vi "HitrapGUI.HTLE_Main.vi"() -> ()   [LabVIEW 2014, in "HitrapGUI.lvlib"]
uses:
  HitrapGUI.lvlib
  CSlibraries/GUILib/GUILib.userEventsMainType.ctl
  CSlibraries-extern/DimLVEvent/DimIndicators/DimIndicators.anyType.ctl
  CSlibraries/UtilityLib/UtilityLib.lvlib
  CSlibraries-extern/DimLVEvent/DimIndicators/DimIndicators.lvlib
  CS_Core/CSSystem/CSSystemLib/CSSystemLib.lvlib
  CS_Core/GUIs/GOGControllerGUI/GOGControllerGUI.lvlib
  CSlibraries/GUILib/GUILib.lvlib
panel:
  in  "TR7":bool
  out "subSystem6State":string
  out "subSystem6StateQuality":string
  in  "TR6-UpperPart":bool
  in  "TR6-LowerPart":bool
  out "subSystem5State":string
  out "subSystem5StateQuality":string
  out "subSystem4State":string
  out "subSystem4StateQuality":string
  in  "TR6BT1":bool
  out "subSystem3State":string
  out "subSystem3StateQuality":string
  in  "TR5":bool
  out "subSystem2State":string
  out "subSystem2StateQuality":string
  in  "NoGUI":bool
  out "subSystem1State":string
  out "subSystem1StateQuality":string
  in  "iniData":string
  in  "subControllersIgnoredDIM":T1
  in  "stop":bool
  in  "userEvent":refnum<user-event>
  # "HITRAP_LE"
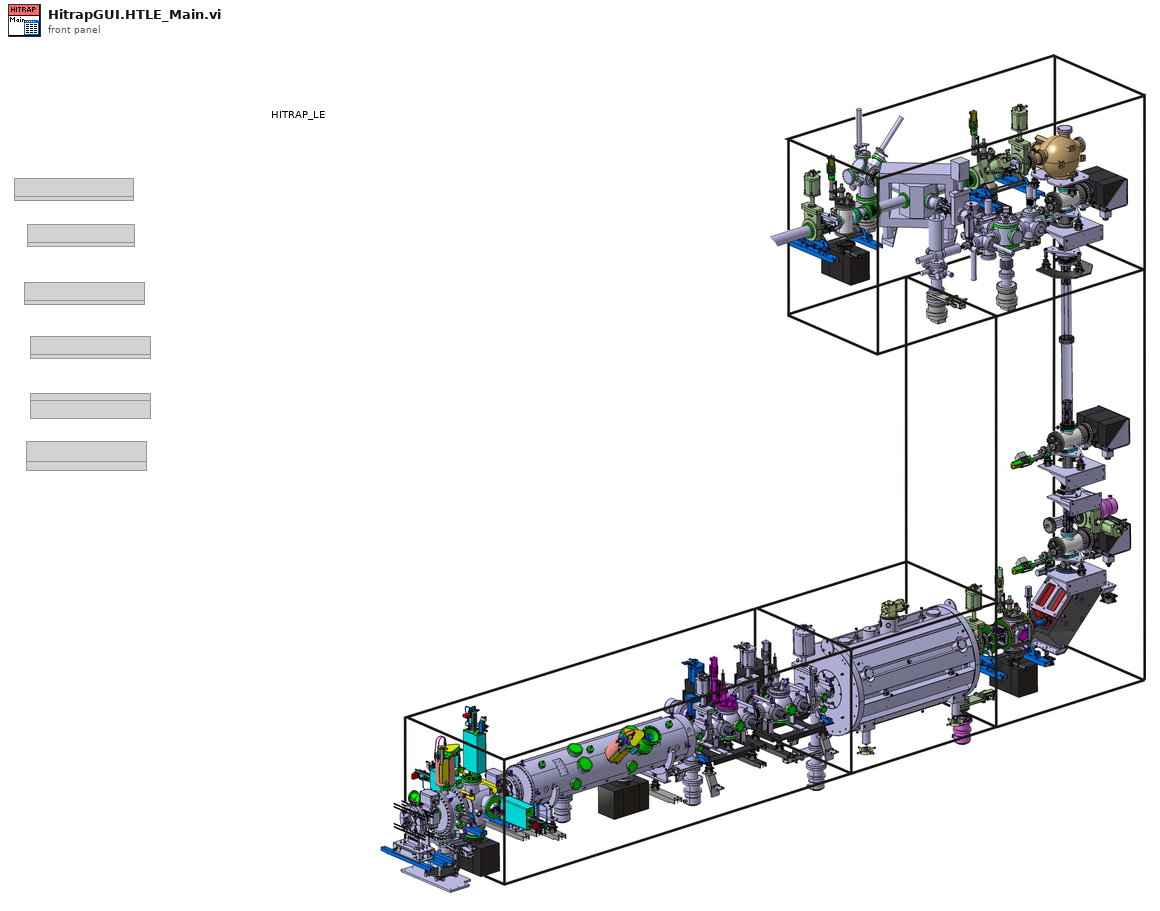
[diagram p1: front panel]
types:
  T1 = typedef "DimIndicators.lvlib/DimIndicators.anyType.ctl" = cluster{"data":string, "no link":bool, "quality":i32, "timeStamp":dbl}
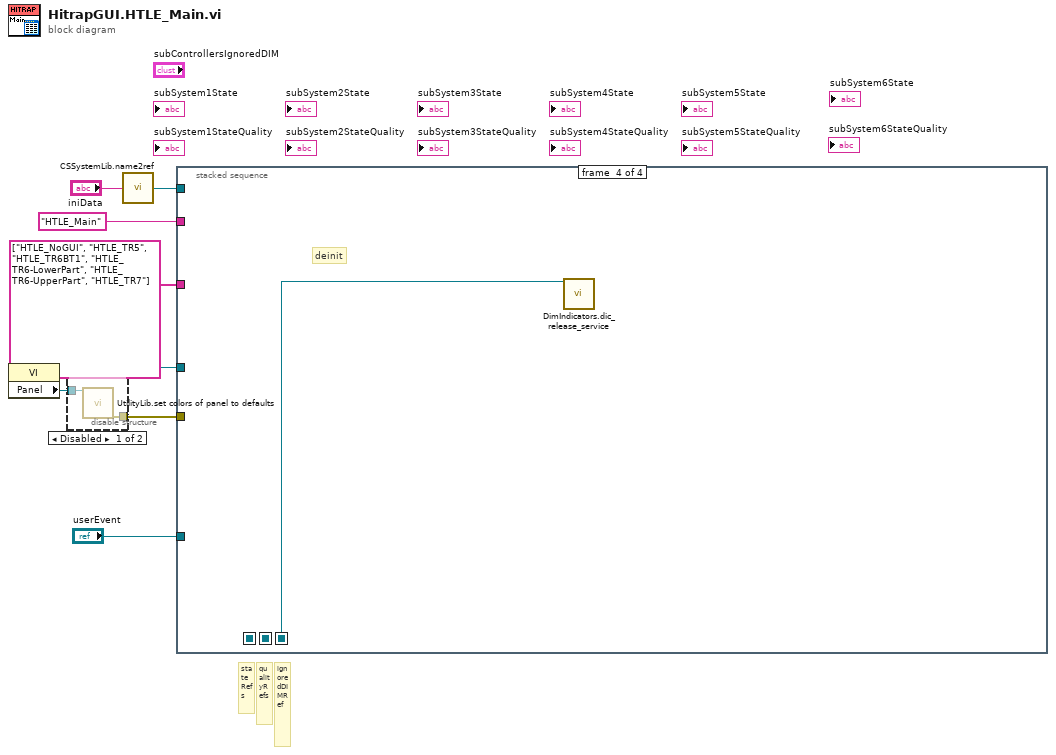
[diagram p0: block diagram]
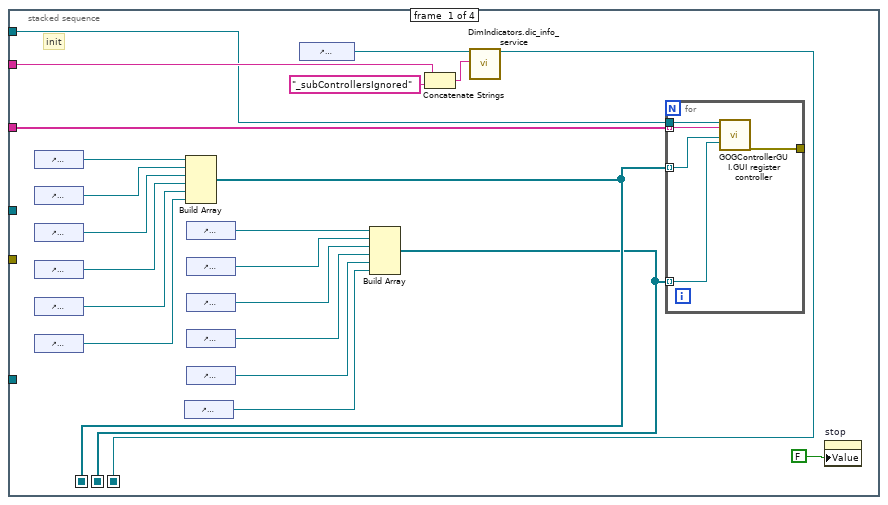
[diagram p3: hidden frame]
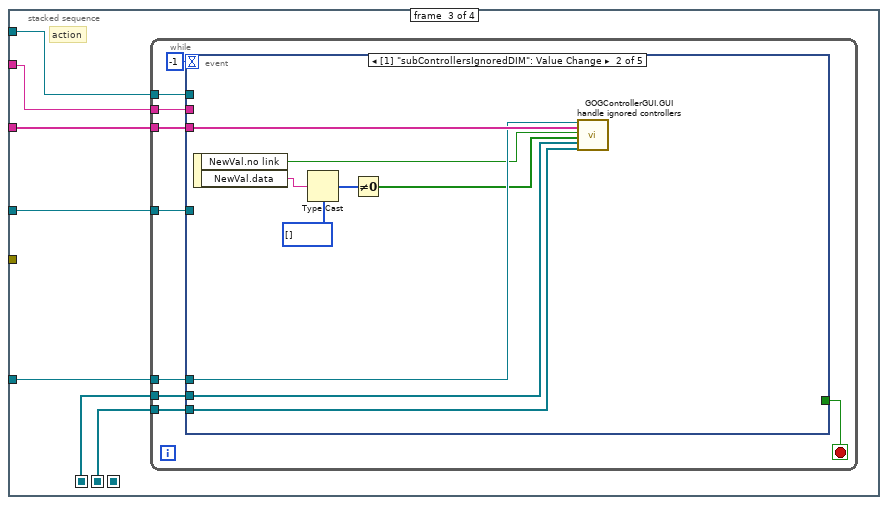
[diagram p5: hidden frame]
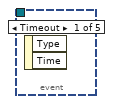
[diagram p6: hidden frame]
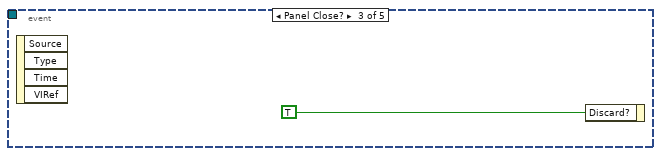
[diagram p7: hidden frame]
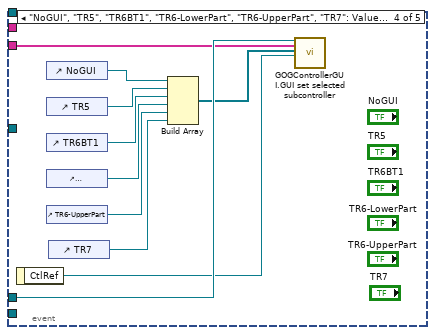
[diagram p8: hidden frame]
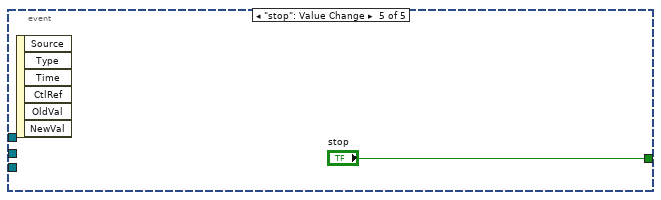
[diagram p9: hidden frame]
diagram:
  # "qualityRefs"
  # "ignoredDIMRef"
  # "stateRefs"
  n1 = property class="VI"() -> (reference out=w6:refnum<vi>, "Panel"=w7:refnum<vi>)  [unwired: 2 in, 1 out]
  n2 = disable-structure shown="Disabled" {
    disable-tunnel: w7 -> [w10 _]
    disable-tunnel: [w9 _] -> w4
    frame Disabled {
      n3 = call "UtilityLib.set colors of panel to defaults.vi"("Front Panel"=w10) -> ("error out"=w9:errorcluster)  [unwired: 18 in]
    }
    frame Enabled {
    }
  }
  n4 = call "CSSystemLib.name2ref.vi"("name"="iniData") -> ("obj refnum"=w1:refnum<vi>)
  n5 = stacked-sequence {
    seq-local: [w25 _ _ _] -> [_ _ _ w75]
    seq-local: [w26 _ _ _] -> [_ _ w41 _]
    seq-local: [w21 _ _ _] -> [_ _ w38 _]
    tunnel: "userEvent" -> [_ _ w44 _]
    tunnel: w6 -> [_ _ w43 _]
    tunnel: string[] ["HTLE_NoGUI", "HTLE_TR5", "HTLE_TR6BT1", "HTLE_TR6-LowerPart", "HTLE_TR6-UpperPart", "HTLE_TR7"] -> [w30 _ w42 _]
    tunnel: w4 -> [_ _ _ _]
    tunnel: "HTLE_Main" -> [w23 _ w40 _]
    tunnel: w1 -> [w22 _ w39 _]
    frame #0 {
      # "init"
      n6 = control-ref of="subSystem1State"() -> (w31:refnum<vi>)
      n7 = control-ref of="subSystem2State"() -> (w20:refnum<vi>)
      n8 = control-ref of="subSystem3State"() -> (w18:refnum<vi>)
      n9 = control-ref of="subSystem4State"() -> (w16:refnum<vi>)
      n10 = control-ref of="subSystem5State"() -> (w15:refnum<vi>)
      n11 = control-ref of="subSystem6State"() -> (w12:refnum<vi>)
      n12 = control-ref of="subSystem6StateQuality"() -> (w11:refnum<vi>)
      n13 = Build Array(w31, w20, w18, w16, w15, w12) -> (w26:refnum<vi>[])
      n14 = control-ref of="subSystem1StateQuality"() -> (w24:refnum<vi>)
      n15 = control-ref of="subSystem2StateQuality"() -> (w19:refnum<vi>)
      n16 = control-ref of="subSystem3StateQuality"() -> (w17:refnum<vi>)
      n17 = control-ref of="subSystem4StateQuality"() -> (w14:refnum<vi>)
      n18 = control-ref of="subSystem5StateQuality"() -> (w13:refnum<vi>)
      n19 = control-ref of="subControllersIgnoredDIM"() -> (w27:refnum<vi>)
      n20 = Build Array(w24, w19, w17, w14, w13, w11) -> (w21:refnum<vi>[])
      n21 = Concatenate Strings(w23, "_subControllersIgnored" ("string")) -> (w28:string)
      n22 = call "DimIndicators.dic_info_service.vi"("controlRef"=w27, "serviceName"=w28) -> ("controlRef out"=w25:refnum<vi>)  [unwired: 16 in, 1 out]
      n23 = for {
        tunnel: w26 -> [w37] mode=indexing
        tunnel: w30 -> [w35] mode=indexing
        tunnel: w21 -> [w34] mode=indexing
        tunnel: w22 -> [w36]
        tunnel: [w33] -> _
        n24 = call "GOGControllerGUI.GUI register controller.vi"("i ref in"=w36, "controllerName"=w35, "subSystemState"=w37, "subSystemStateQuality"=w34) -> ("error out"=w33:errorcluster)  [unwired: 14 in, 1 out]
      }
      n25 = property on="stop" class="Bool (strict)"("Value"=FALSE ("stop")) -> ()  [unwired: 2 in, 2 out]
    }
    frame #1 {
      # "more init"
    }
    frame #2 {
      # "action"
      n26 = while {
        tunnel: w44 -> [w53]
        tunnel: w43 -> [w52]
        tunnel: w42 -> [w50]
        tunnel: w41 -> [w49]
        tunnel: w39 -> [w47]
        tunnel: w40 -> [w46]
        tunnel: w38 -> [w45]
        stop <- w51 stop-if-true
        n27 = event shown="[1] \"subControllersIgnoredDIM\": Value Change" {
          selector: _ -> [_ _ _ _ _]
          dyn-events: _ -> [_ _ _ _ _]
          timeout: -1 -> [_ _ _ _ _]
          tunnel: w53 -> [_ w61 _ w73 _]
          tunnel: w52 -> [_ _ _ _ _]
          tunnel: [_ _ _ _ "stop"] -> w51
          tunnel: w50 -> [_ w62 _ w72 _]
          tunnel: w49 -> [_ w55 _ _ _]
          tunnel: w47 -> [_ _ _ _ _]
          tunnel: w46 -> [_ _ _ _ _]
          tunnel: w45 -> [_ w54 _ _ _]
          event Timeout {
            n28 = event-data() -> ()  [unwired: 1 in, 2 out]
          }
          event Value Change {
            n29 = event-data() -> ("NewVal.no link"=w60:bool, "NewVal.data"=w59:string)  [unwired: 1 in]
            n30 = Type Cast(type=i16[] [] ("Array"), x=w59) -> (*(type *) &x=w57:i16[])
            n31 = Not Equal To 0?(x=w57) -> (x != 0?=w56:bool[])
            n32 = call "GOGControllerGUI.GUI handle ignored controllers.vi"("userEvent"=w61, "controllerNames"=w62, "NOLINK"=w60, "controllersIgnored"=w56, "stateRefs"=w55, "qualityRefs"=w54) -> ()  [unwired: 14 in]
          }
          event Panel Close? {
            n33 = event-data() -> ()  [unwired: 1 in, 4 out]
            n34 = event-data("Discard?"=TRUE) -> ()  [unwired: 1 in, 1 out]
          }
          event "NoGUI", "TR5", "TR6BT1", "TR6-LowerPart", "TR6-UpperPart", "TR7": Value Change {
            n35 = event-data() -> ("CtlRef"=w69:refnum<vi>)  [unwired: 1 in]
            n36 = control-ref of="NoGUI"() -> (w70:refnum<vi>)
            n37 = control-ref of="TR5"() -> (w68:refnum<vi>)
            n38 = control-ref of="TR6BT1"() -> (w67:refnum<vi>)
            n39 = control-ref of="TR6-LowerPart"() -> (w66:refnum<vi>)
            n40 = control-ref of="TR6-UpperPart"() -> (w65:refnum<vi>)
            n41 = control-ref of="TR7"() -> (w64:refnum<vi>)
            n42 = Build Array(w70, w68, w67, w66, w65, w64) -> (w71:refnum<vi>[])
            n43 = call "GOGControllerGUI.GUI set selected subcontroller.vi"("userEvent"=w73, "controllerNames"=w72, "controllerRefs"=w71, "controllerRef"=w69) -> ()  [unwired: 16 in]
          }
          event "stop": Value Change {
            n44 = event-data() -> ()  [unwired: 1 in, 6 out]
          }
        }
      }
    }
    frame #3 {
      # "deinit"
      n45 = call "DimIndicators.dic_release_service.vi"("controlRef"=w75) -> ()  [unwired: 18 in, 1 out]
    }
  }
